vi "calculate_trajectory_bounding_box.vi"(8 "error in (no error)":errorcluster, 11 "DL090202ScanHead in":refnum<class "ScanHeadDL090202.lvclass">) -> (0 "error out":errorcluster, 2 "bounding box":refnum<class "Box.lvclass">, 3 "DL090202ScanHead out":refnum<class "ScanHeadDL090202.lvclass">)   [LabVIEW 2010, in "ScanHeadDL090202.lvclass"]
uses:
  ScanHeadDL090202.lvclass
  common/classes/Box/Box/Box.lvclass
  ScanHeadDL090202.lvclass/ScanHeadDL090202.ctl
  SignalWriter/GenericSignalWriter/GenericSignalWriter/GenericSignalWriter.lvclass
  Objective/GenericObjective/GenericObjective/GenericObjective.lvclass
  common/classes/ErrorController/ErrorController/class_data.vi
  common/classes/SpaceVector/SpaceVector/SpaceVector.lvclass
  common/classes/ErrorController/ErrorController/ErrorController.lvclass
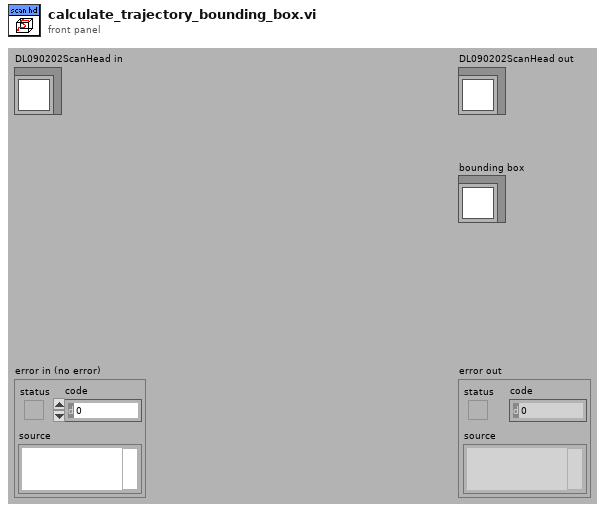
[diagram p1: front panel]
types:
  T1 = cluster{"[0]":dbl[unit], "[1]":dbl[unit], "[2]":dbl[unit]}
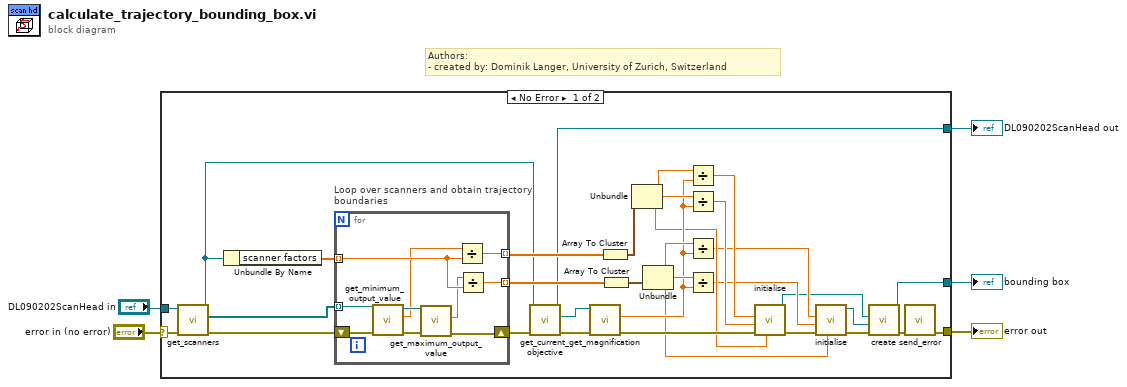
[diagram p0: block diagram]
diagram:
  # "Authors: \n- created by: Dominik Langer, University of Zurich, Switzerland"
  n1 = case shown="No Error" "error in (no error)" {
    selector: "error in (no error)" -> [w12 w50]
    tunnel: [w6 w50] -> w4
    tunnel: [w14 w49] -> w2
    tunnel: "DL090202ScanHead in" -> [w9 w49]
    tunnel: [w17 _] -> w1
    frame No Error {
      n2 = call-dynamic "get_scanners.vi"("error in (no error)"=w12, "DL090202ScanHead.lvclass in"=w9) -> ("error out"=w11:errorcluster, "scanners"=w10:refnum<class "GenericSignalWriter.lvclass">[], "DL090202ScanHead.lvclass out"=w8:refnum<class "ScanHeadDL090202.lvclass">)  [unwired: 7 in]
      n3 = Unbundle By Name(w8) -> ("scanner factors"=w38:dbl[unit][])
      n4 = for "Loop over scanners and obtain trajectory boundaries" {
        tunnel: w10 -> [w46] mode=indexing
        shift-right: [w39] -> w16
        shift-left: w11 -> [w48]
        tunnel: w38 -> [w44] mode=indexing
        tunnel: [w41] -> w30 mode=indexing
        tunnel: [w40] -> w31 mode=indexing
        n5 = call-dynamic "get_minimum_output_value.vi"("error in (no error)"=w48, "GenericWriteSignals.lvclass in"=w46) -> ("error out"=w47:errorcluster, "minimum output value"=w43:dbl, "GenericWriteSignals.lvclass out"=w45:refnum<class "GenericSignalWriter.lvclass">)  [unwired: 7 out]
        n6 = call-dynamic "get_maximum_output_value.vi"("error in (no error)"=w47, "GenericWriteSignals.lvclass in"=w45) -> ("error out"=w39:errorcluster, "maximum output value"=w42:dbl)  [unwired: 8 out]
        n7 = Divide(x=w43, y=w44) -> (x/y=w40:dbl[unit])
        n8 = Divide(x=w42, y=w44) -> (x/y=w41:dbl[unit])
      }
      n9 = call-dynamic "get_current_objective.vi"("error in (no error)"=w16, "GenericPlugin in"=w8) -> ("error out"=w15:errorcluster, "current objective"=w13:refnum<class "GenericObjective.lvclass">, "GenericPlugin out"=w14:refnum<class "ScanHeadDL090202.lvclass">)  [unwired: 7 in]
      n10 = call-dynamic "get_magnification.vi"("error in (no error)"=w15, "GenericObjective in"=w13) -> ("error out"=w28:errorcluster, "magnification"=w29:dbl)  [unwired: 5 in, 3 out]
      n11 = Array To Cluster(array=w31) -> (cluster=w37:T1)
      n12 = Array To Cluster(array=w30) -> (cluster=w36:T1)
      n13 = Unbundle(w37) -> ("[0]"=w35:dbl[unit], "[1]"=w34:dbl[unit], "[2]"=w26:dbl[unit])
      n14 = Unbundle(w36) -> ("[0]"=w33:dbl[unit], "[1]"=w32:dbl[unit], "[2]"=w21:dbl[unit])
      n15 = Divide(x=w35, y=w29) -> (x/y=w24:dbl[unit])
      n16 = Divide(x=w34, y=w29) -> (x/y=w25:dbl[unit])
      n17 = Divide(x=w33, y=w29) -> (x/y=w23:dbl[unit])
      n18 = Divide(x=w32, y=w29) -> (x/y=w22:dbl[unit])
      n19 = call "initialise.vi"("z"=w26, "error in (no error)"=w28, "y"=w25, "x"=w24) -> ("error out"=w27:errorcluster, "SpaceVector out"=w19:refnum<class "SpaceVector.lvclass">)  [unwired: 6 out]
      n20 = call "initialise.vi"("z"=w21, "error in (no error)"=w27, "y"=w22, "x"=w23) -> ("error out"=w20:errorcluster, "SpaceVector out"=w18:refnum<class "SpaceVector.lvclass">)  [unwired: 6 out]
      n21 = call "create.vi"("error in (no error)"=w20, "maximum"=w18, "minimum"=w19) -> ("error out"=w7:errorcluster, "Box out"=w17:refnum<class "Box.lvclass">)  [unwired: 7 out]
      n22 = call "send_error.vi"("error in (no error)"=w7) -> ("error out"=w6:errorcluster)  [unwired: 10 in]
    }
    frame Error {
    }
  }
  "error out" <- w4
  "DL090202ScanHead out" <- w2
  "bounding box" <- w1
